vi "Initialize All AI Channels and TaskRefs.vi"(0 "DAQ":refnum<class "DAQ.lvclass">, 1 "offsets":T4, 3 "AI Settings[]":T1[](array[typedef]), 5 "DAQNode Dict":T5, 7 "AI Tasks":T6[](array[typedef]) {"AI Channels"."Force Bridge"."scaling information"."physical units" items=["Newtons"=15875, "Pounds"=15876, "kgf"=15877]; "AI Channels"."Force Bridge"."scaling information"."electrical units" items=["Volts/Volt"=15896, "mVolts/Volt"=15897]; "AI Channels"."Force Bridge"."bridge information"."voltage excitation source" items=["Internal"=10200, "External"=10167]; "AI Channels"."Force Bridge"."bridge information"."bridge configuration" items=["Full Bridge"=10182, "Half Bridge"=10187, "Quarter Bridge"=10270]; "AI Channels"."Conversion"."ScaleOffset" format="%.3f"; "AI Channels"."Conversion"."MinEngUnit" format="%.3f"; "AI Channels"."Conversion"."MaxEngUnit" format="%.3f"; "AI Channels"."Conversion"."MinSignal" format="%.3f"; "AI Channels"."Conversion"."MaxSignal" format="%.3f"; "AI Channels"."Terminal Configuration" items=["default"=-1, "RSE"=10083, "NRSE"=10078, "Differential"=10106, "Pseudodifferential"=12529]}, 11 "error in":errorcluster, 14 "Simulate":bool) -> (4 "DAQ out":refnum<class "DAQ.lvclass">, 6 "DAQNode Dict out":T5, 8 "DAQmxTaskAI[]":refnum<k21>[](array[refnum]), 10 "AI TaskNames":string[](array[string]), 15 "error out":errorcluster)   [LabVIEW 2017, in "DAQ.lvclass"]
doc: "Developed by Kevin Thompson\nkevin@thompsonengineering.net\n\nCopyright 2015\nThompson Engineering, LLC"
uses:
  DAQ.lvclass
  DataTypes/TD AI Task--cluster.ctl
  DataTypes/TD AI Channel--cluster.ctl
  DataTypes/TD DataValueConversion--cluster.ctl
  DataTypes/TD AI DAQ Type--enum.ctl
  DataTypes/TD AI Force Bridge--cluster.ctl
  <vilib>/TELLC/Dynamic CVT API/TD Dynamic CVT DVR--ref.ctl
  DataTypes/offsets cluster.ctl
  DataTypes/TD AI Instrument Settings--cluster.ctl
  DataTypes/TD AI InstSettings--cluster.ctl
  Process/ProcessSupport/TD SimAI Ranges--cluster.ctl
  DAQ.lvclass/DAQ.ctl
  Accessors/Set AI IONames.vi
  Accessors/Set AI SchemNames.vi
  Accessors/Set AI Settings.vi
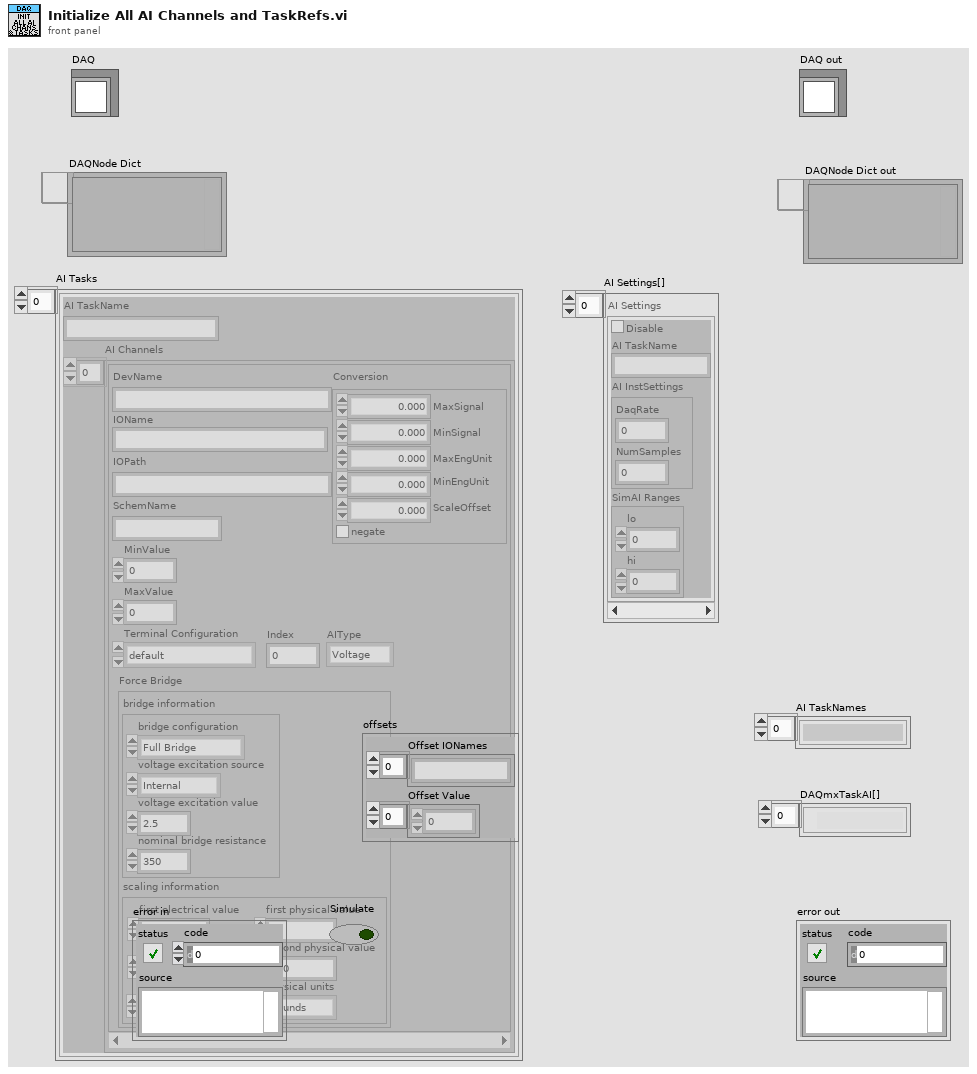
[diagram p1: front panel]
types:
  T1 = typedef "DAQ.lvclass/TD AI Instrument Settings--cluster.ctl" = cluster{"Disable":bool, "AI TaskName":string, "AI InstSettings":T2, "SimAI Ranges":T3}
  T2 = typedef "DAQ.lvclass/TD AI InstSettings--cluster.ctl" = cluster{"DaqRate":dbl, "NumSamples":i32}
  T3 = typedef "DAQ.lvclass/TD SimAI Ranges--cluster.ctl" = cluster{"lo":dbl, "hi":dbl}
  T4 = typedef "DAQ.lvclass/offsets cluster.ctl" = cluster{"Offset IONames":string[], "Offset Value":dbl[]}
  T5 = typedef "TD Dynamic CVT DVR--ref.ctl" = refnum<data-value>
  T6 = typedef "DAQ.lvclass/TD AI Task--cluster.ctl" = cluster{"AI TaskName":string, "AI Channels":T7[]}
  T7 = typedef "DAQ.lvclass/TD AI Channel--cluster.ctl" = cluster{"DevName":string, "IOName":string, "IOPath":string, "SchemName":string, "MinValue":dbl, "MaxValue":dbl, "Terminal Configuration":i32, "Index":i32, "Conversion":T8, "AIType":T9, "Force Bridge":T10}
  T8 = typedef "DAQ.lvclass/TD DataValueConversion--cluster.ctl" = cluster{"MaxSignal":dbl, "MinSignal":dbl, "MaxEngUnit":dbl, "MinEngUnit":dbl, "ScaleOffset":dbl, "negate":bool}
  T9 = typedef "DAQ.lvclass/TD AI DAQ Type--enum.ctl" = enum16{"Voltage", "Current", "Strain Gage", "Force Bridge"}
  T10 = typedef "DAQ.lvclass/TD AI Force Bridge--cluster.ctl" = cluster{"bridge information":cluster{"bridge configuration":i32, "voltage excitation source":i32, "voltage excitation value":dbl, "nominal bridge resistance":dbl}, "scaling information":cluster{"first electrical value":dbl, "second electrical value":dbl, "electrical units":i32, "first physical value":dbl, "second physical value":dbl, "physical units":i32}}
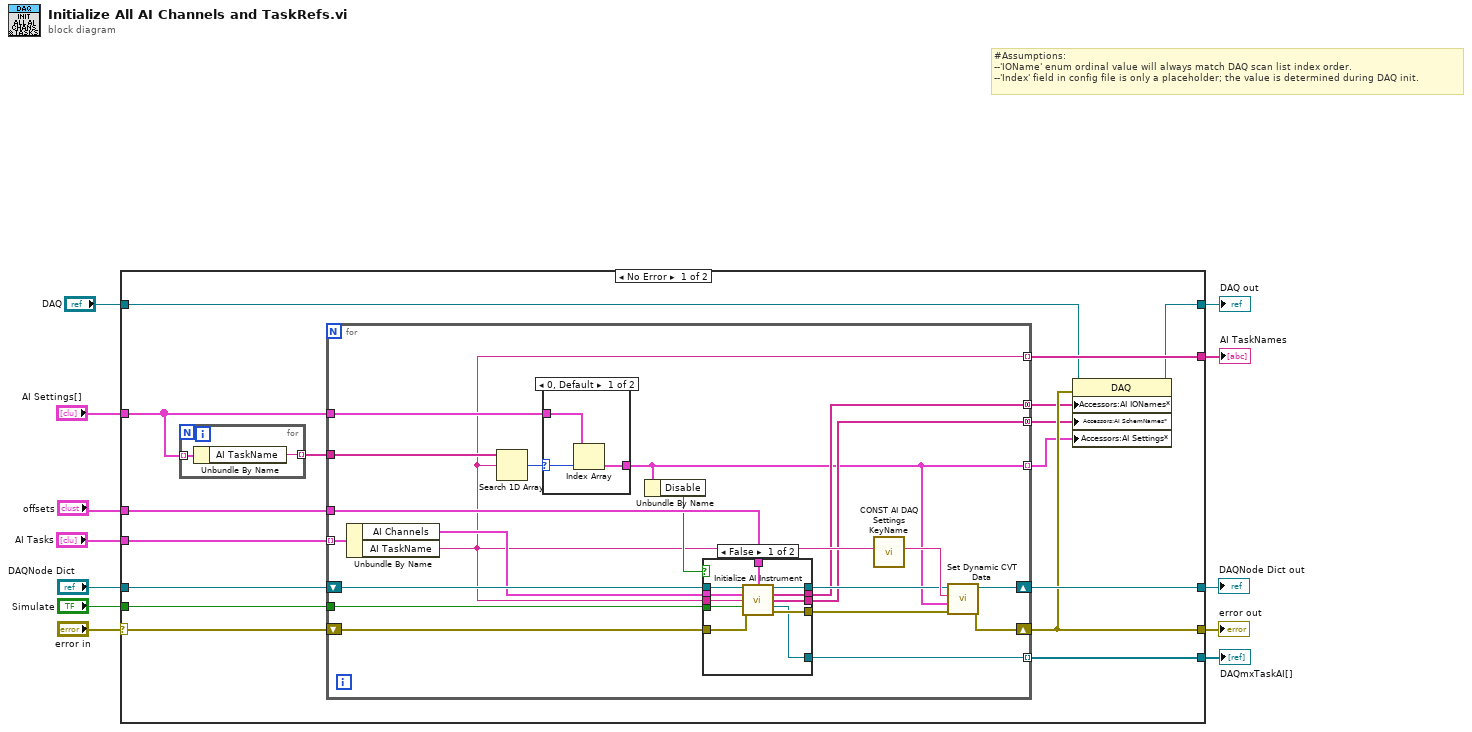
[diagram p0: block diagram]
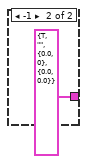
[diagram p3: hidden frame]
diagram:
  # "#Assumptions:\n--'IOName' enum ordinal value will always match DAQ scan list index order.\n--'Index' field in config file is only a placeholder; the value is determined during DAQ init."
  n1 = case shown="No Error" "error in" {
    selector: "error in" -> [w26 w70]
    tunnel: "AI Tasks" -> [w23 _]
    tunnel: "DAQNode Dict" -> [w28 w69]
    tunnel: [w17 w70] -> w10
    tunnel: [w25 w69] -> w4
    tunnel: "Simulate" -> [w27 _]
    tunnel: "offsets" -> [w22 _]
    tunnel: [w24 _] -> w6
    tunnel: "AI Settings[]" -> [w20 _]
    tunnel: [w19 _] -> w3
    tunnel: "DAQ" -> [w14 w68]
    tunnel: [w18 w68] -> w1
    frame No Error {
      n2 = for {
        tunnel: [w67] -> w21 mode=indexing
        tunnel: w20 -> [w66] mode=indexing
        n3 = Unbundle By Name(w66) -> ("AI TaskName"=w67:string)
      }
      n4 = for {
        tunnel: w27 -> [w47]
        tunnel: [w40] -> w24 mode=indexing
        shift-right: [w44] -> w25
        shift-left: w28 -> [w48]
        shift-right: [w45] -> w17
        shift-left: w26 -> [w46]
        tunnel: w23 -> [w39] mode=indexing
        tunnel: w22 -> [w37]
        tunnel: w21 -> [w36]
        tunnel: w20 -> [w34]
        tunnel: [w32] -> w19 mode=indexing
        tunnel: [w31] -> w16 mode=concatenating
        tunnel: [w30] -> w15 mode=concatenating
        tunnel: [w29] -> w13 mode=indexing
        n5 = Unbundle By Name(w39) -> ("AI Channels"=w38:T7[], "AI TaskName"=w32:string)
        n6 = Search 1D Array(1D array=w36, element=w32) -> (index of element=w35:i32)  [unwired: 1 in]
        n7 = case shown="0, Default" w35 {
          selector: w35 -> [w63 _]
          tunnel: [w64 T1 {"Disable"=TRUE, "AI TaskName"="", "AI InstSettings"={"DaqRate"=0.0, "NumSamples"=0}, "SimAI Ranges"={"lo"=0.0, "hi"=0.0}} ("AI Settings")] -> w29
          tunnel: w34 -> [w62 _]
          frame 0, Default {
            n8 = Index Array(array=w62, index=w63) -> (element=w64:T1)
          }
          frame -1 {
          }
        }
        n9 = Unbundle By Name(w29) -> ("Disable"=w33:bool)
        n10 = case shown="False" w33 {
          tunnel: w48 -> [w59 w61]
          tunnel: w47 -> [w58 _]
          tunnel: w46 -> [w57 w60]
          tunnel: [w56 w61] -> w42
          tunnel: [w55 w60] -> w41
          tunnel: [w51 _] -> w40
          tunnel: w38 -> [w54 _]
          tunnel: w37 -> [w53 _]
          tunnel: w32 -> [w52 _]
          tunnel: [w50 _] -> w31
          tunnel: [w49 _] -> w30
          frame False {
            n11 = call "Initialize AI Instrument.vi"("DAQNode Dict"=w59, "offsets"=w53, "AI Channels"=w54, "AI TaskName"=w52, "Simulate"=w58, "error in (no error)"=w57) -> ("DAQNode Dict out"=w56:T5, "AI IONames"=w50:string[], "AI SchemNames"=w49:string[], "DAQmx Task AI"=w51:refnum<k21>, "error out"=w55:errorcluster)  [unwired: 5 in]
          }
          frame True {
          }
        }
        n12 = call "CONST AI DAQ Settings KeyName.vi"("AI TaskName"=w32) -> ("AI DAQ Settings (KeyName)"=w43:string)  [unwired: 10 in]
        n13 = call <vilib>:"Set Dynamic CVT Data.vi"("error in (no error)"=w41, "value"=w29, "DataName"=w43, "dCVT DVR"=w42) -> ("error out"=w45:errorcluster, "dCVT DVR out"=w44:T5)  [unwired: 5 in, 1 out]
      }
      n14 = property class="DAQ"(reference=w14, error in=w17, "Accessors:AI IONames*"=w16, "Accessors:AI SchemNames*"=w15, "Accessors:AI Settings*"=w13) -> (reference out=w18:refnum<class "DAQ.lvclass">)  [unwired: 1 out]
    }
    frame Error {
    }
  }
  "error out" <- w10
  "DAQNode Dict out" <- w4
  "DAQmxTaskAI[]" <- w6
  "AI TaskNames" <- w3
  "DAQ out" <- w1
